vi "Sequence Array Info.vi"(10 "Seq In":T4 {"Image Acquisition Parameters Out"."Z Steps Size (um)" min=0.0; "Image Acquisition Parameters Out"."Number of Z Steps" min=1; "Image Acquisition Parameters Out"."Frames Accumulations" min=1; "Image Acquisition Parameters Out"."Frames Per Capture" min=1; "Image Acquisition Parameters Out"."Line Accumulations" min=1; "Image Acquisition Parameters Out"."Image Format" items=["64 x 64"=64, "128 x 128"=128, "256 x 256"=256, "512 x 512"=512, "1024 x 1024"=1024, "2048 x 2048"=2048]; "Detectors Parameters Out"."405 Power (0-5V)" min=0.0 max=5.0}, 11 "Action":enum16{"Add", "Remove", "Update", "Clear"}(ring)) -> (3 "Seq Array Out":T5(array[cluster]) {"Image Acquisition Parameters Out"."Z Steps Size (um)" min=0.0; "Image Acquisition Parameters Out"."Number of Z Steps" min=1; "Image Acquisition Parameters Out"."Frames Accumulations" min=1; "Image Acquisition Parameters Out"."Frames Per Capture" min=1; "Image Acquisition Parameters Out"."Line Accumulations" min=1; "Image Acquisition Parameters Out"."Image Format" items=["64 x 64"=64, "128 x 128"=128, "256 x 256"=256, "512 x 512"=512, "1024 x 1024"=1024, "2048 x 2048"=2048]; "Detectors Parameters Out"."405 Power (0-5V)" min=0.0 max=5.0})   [LabVIEW 2016]
uses:
  Type Defs/Image Acquisition Parameters.ctl
  Laser Controls.ctl
  Detectors.ctl
panel:
  # "Copyright (C) 2020 Edward S Allgeyer\n\nRedistribution and use in source and binary forms, with or without\nmodification, are permitted provided that the following conditions\nare met:\n\n1. Redistributions of source code must retain the above copyright\n   notice, this list of conditions and the following disclaimer.\n\n2. Redistributions in binary form must reproduce the above copyright\n   notice, this list of conditions and the following disclaimer in\n   the documentation and/or other materials provided with the\n   distribution.\n\n3. Neither the name of the copyright holder nor the names of its\n   contributors may be used to endorse or promote products derived\n   from this software without specific prior written permission.\n\nTHIS SOFTWARE IS PROVIDED BY THE COPYRIGHT HOLDERS AND CONTRIBUTORS\n\"AS IS\" AND ANY EXPRESS OR IMPLIED WARRANTIES, INCLUDING, BUT NOT\nLIMITED TO, THE IMPLIED WARRANTIES OF MERCHANTABILITY AND FITNESS\nFOR A PARTICULAR PURPOSE ARE DISCLAIMED. IN NO EVENT SHALL THE\nCOPYRIGHT HOLDER OR CONTRIBUTORS BE LIABLE FOR ANY DIRECT, INDIRECT,\nINCIDENTAL, SPECIAL, EXEMPLARY, OR CONSEQUENTIAL DAMAGES (INCLUDING,\nBUT NOT LIMITED TO, PROCUREMENT OF SUBSTITUTE GOODS OR SERVICES;\nLOSS OF USE, DATA, OR PROFITS; OR BUSINESS INTERRUPTION) HOWEVER\nCAUSED AND ON ANY THEORY OF LIABILITY, WHETHER IN CONTRACT, STRICT\nLIABILITY, OR TORT (INCLUDING NEGLIGENCE OR OTHERWISE) ARISING IN\nANY WAY OUT OF THE USE OF THIS SOFTWARE, EVEN IF ADVISED OF THE\nPOSSIBILITY OF SUCH DAMAGE."
  # "XY"
  # "Z"
  # "Length"
  # "Height"
  # "XY"
  # "Z"
  # "Length"
  # "Height"
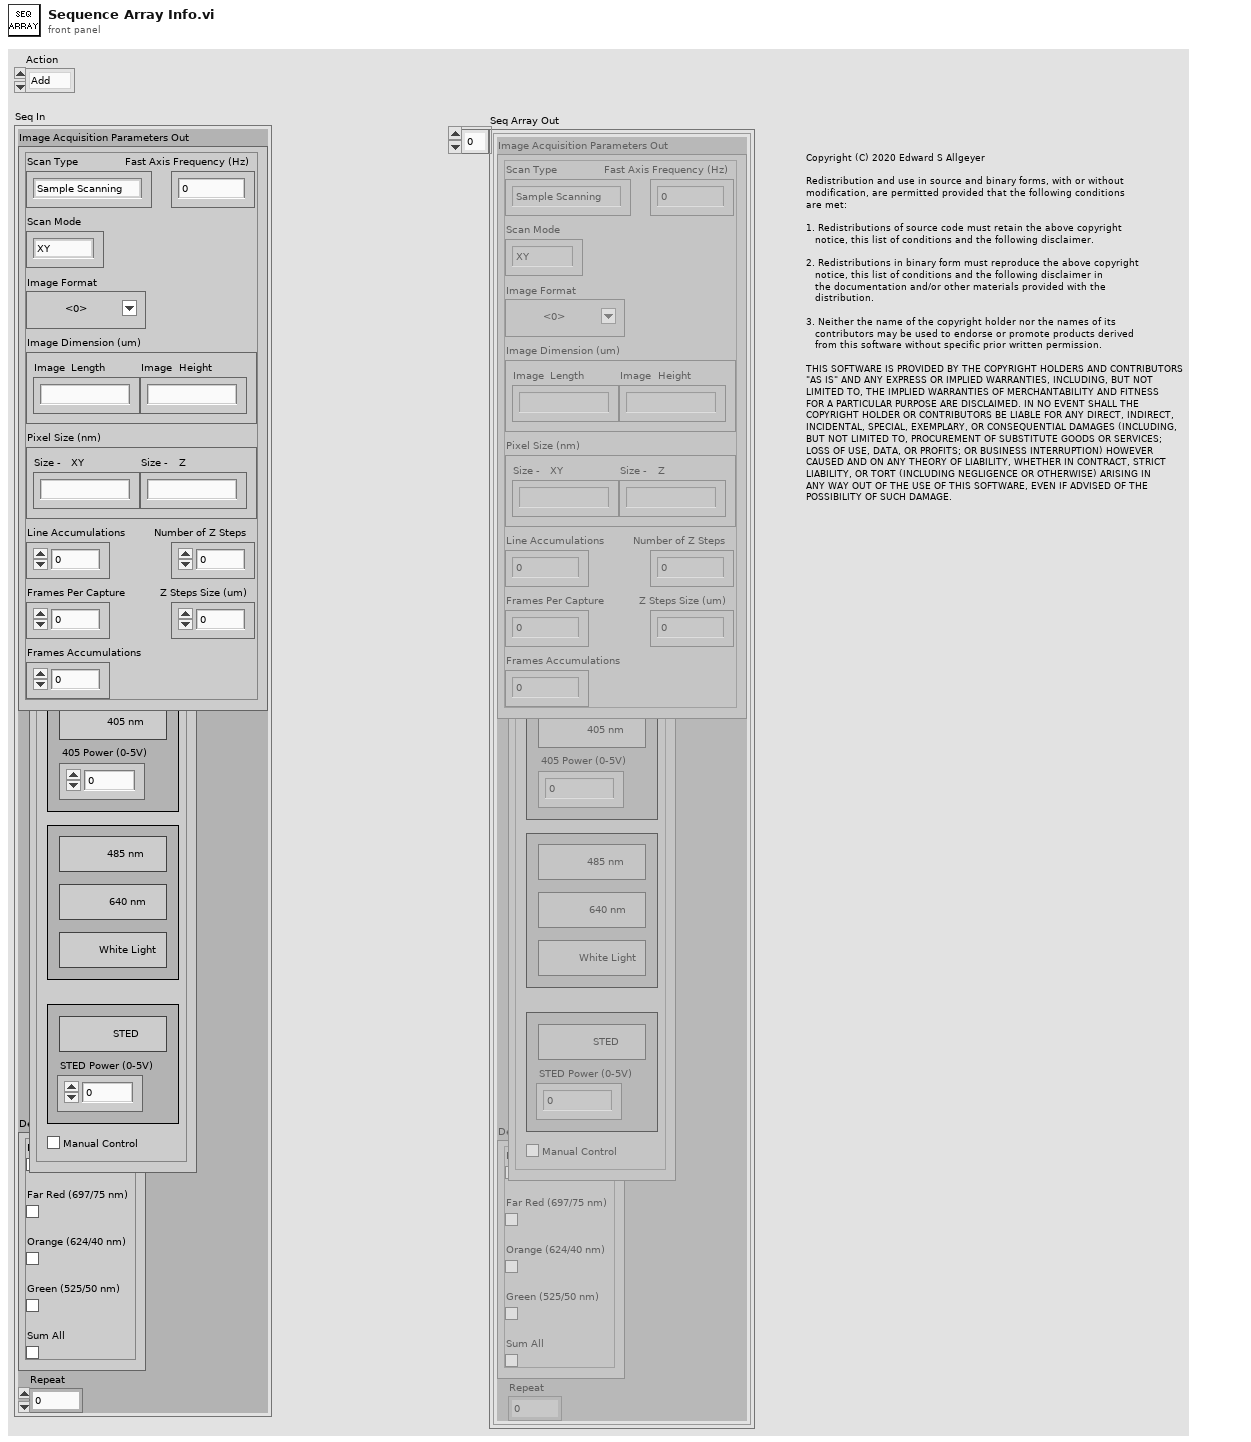
[diagram p1: front panel]
types:
  T1 = typedef "Image Acquisition Parameters.ctl" = cluster{"Scan Type":enum16{"Sample Scanning", "Beam Scanning"}, "Scan Mode":enum16{"XY", "XZ", "YZ", "XYZ"}, "Fast Axis Frequency (Hz)":dbl, "Image Format":u16, "Line Accumulations":u16, "Frames Per Capture":u16, "Frames Accumulations":u16, "Image Dimension (um)":dbl[], "Number of Z Steps":u8, "Z Steps Size (um)":dbl, "Pixel Size (nm)":dbl[]}
  T2 = typedef "Laser Controls.ctl" = cluster{"STED Power (0-5V)":dbl, "STED":bool, "640 nm":bool, "485 nm":bool, "Manual Control":bool, "White Light":bool, "405 nm":bool, "405 Power (0-5V)":dbl}
  T3 = typedef "Detectors.ctl" = cluster{"PMT":bool, "Far Red (697/75 nm)":bool, "Orange (624/40 nm)":bool, "Green (525/50 nm)":bool, "Sum All":bool}
  T4 = cluster{"Image Acquisition Parameters Out":T1, "Detectors Parameters Out":T2, "Detectors Parameters Out":T3, "Repeat":dbl}
  T5 = cluster{"Image Acquisition Parameters Out":T1, "Detectors Parameters Out":T2, "Detectors Parameters Out":T3, "Repeat":dbl}[]
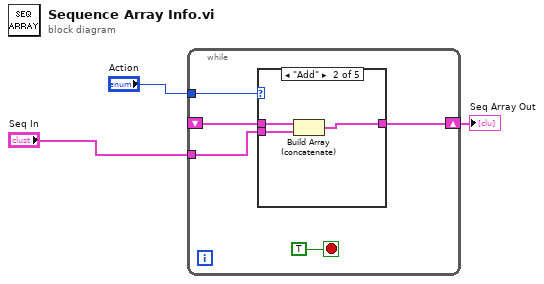
[diagram p0: block diagram]
diagram:
  n1 = while {
    shift-right: [w5] -> w3
    shift-left: _ -> [w7]
    tunnel: "Seq In" -> [w6]
    tunnel: "Action" -> [w4]
    stop <- TRUE stop-if-true
    n2 = case shown="\"Add\"" w4 {
      tunnel: w7 -> [_ w11 _ _ _]
      tunnel: w6 -> [_ w10 _ _ _]
      tunnel: [_ w9 _ _ _] -> w5
      frame "Add", Default {
      }
      frame "Add" {
        n3 = Build Array (concatenate)(w11, w10) -> (w9:T5)
      }
      frame "Remove" {
      }
      frame "Update" {
      }
      frame "Clear" {
      }
    }
  }
  "Seq Array Out" <- w3
